vi "Check if Service Exists.vi"(8 "error in (no error)":errorcluster, 10 "Service in":refnum<class "Service.lvclass">, 11 "Server in":refnum<class "Server.lvclass">) -> (0 "error out":errorcluster, 2 "Service Exists":bool, 3 "Service out":refnum<class "Service.lvclass">)   [LabVIEW 2024, in "Ramses Framework.lvlib" / "Server.lvclass"]
uses:
  Server.lvclass
  Service/Service.lvclass
  Server.lvclass/Server.ctl
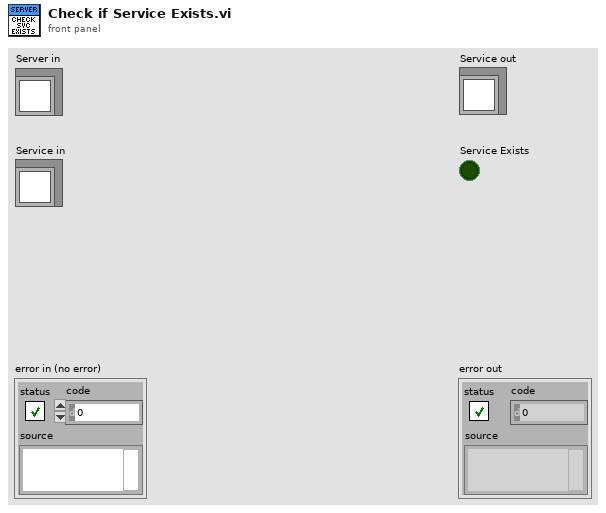
[diagram p1: front panel]
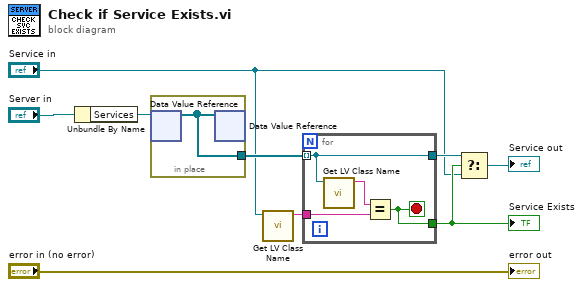
[diagram p0: block diagram]
diagram:
  n1 = Unbundle By Name("Server in") -> ("Services"=w6:refnum<data-value>)
  n2 = in-place {
    in-place-border: [w10] -> w7
    n3 = in-place-dvr #1(w6) -> (w10:refnum<class "Service.lvclass">[])  [unwired: 1 out]
    n4 = in-place-dvr #1(w10) -> ()  [unwired: 2 out]
  }
  n5 = call <vilib>:"Get LV Class Name.vi"("object"="Service in") -> ("class name"=w5:string)  [unwired: 9 in, 1 out]
  n6 = for {
    tunnel: w7 -> [w11] mode=indexing
    tunnel: w5 -> [w13]
    tunnel: [w12] -> w4
    tunnel: [w11] -> w3
    stop <- w12 stop-if-true
    n7 = call <vilib>:"Get LV Class Name.vi"("object"=w11) -> ("class name"=w14:string)  [unwired: 9 in, 1 out]
    n8 = Equal?(x=w14, y=w13) -> (x = y?=w12:bool)
  }
  "Service Exists" <- w4
  n9 = Select(t=w3, s=w4, f="Service in") -> (s? t:f=→"Service out":refnum<class "Service.lvclass">)
  "error out" <- "error in (no error)"
